vi "Get Game Time.vi"(5 "update ui":bool, 7 "Time":refnum<vi>, 8 "error in (no error)":errorcluster, 9 "Pause/Resume":bool, 11 "Application in":refnum<class "Application.lvclass">) -> (0 "error out":errorcluster, 1 "Elapsed":u32, 3 "Stringed Timer Out":string)   [LabVIEW 2021, in "Application.lvclass"]
uses:
  Application.lvclass
  Application.lvclass/Application.ctl
  <userlib>/_OpenG.lib/boolean/boolean.llb/openg_boolean__ogtk.lvlib
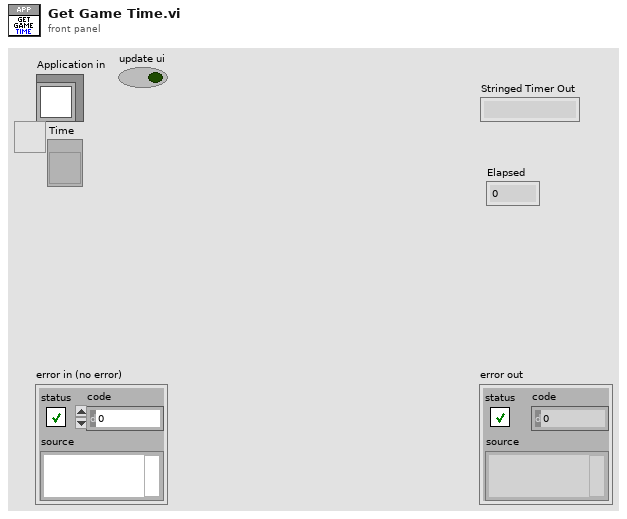
[diagram p1: front panel]
types:
  T1 = cluster{"millisecond timer value":u32, "Elapsed":u32}
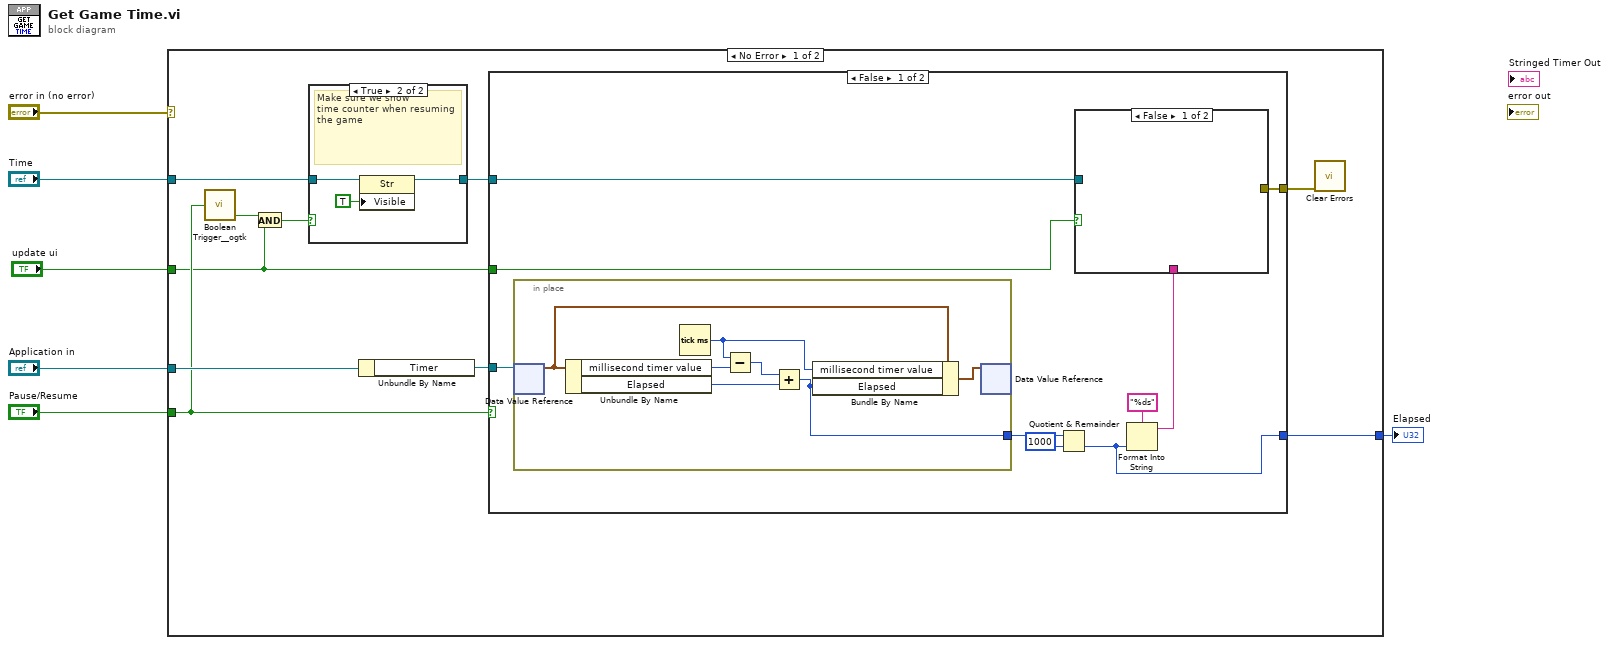
[diagram p0: block diagram]
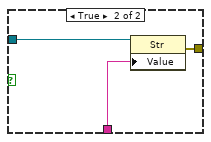
[diagram p3: hidden frame]
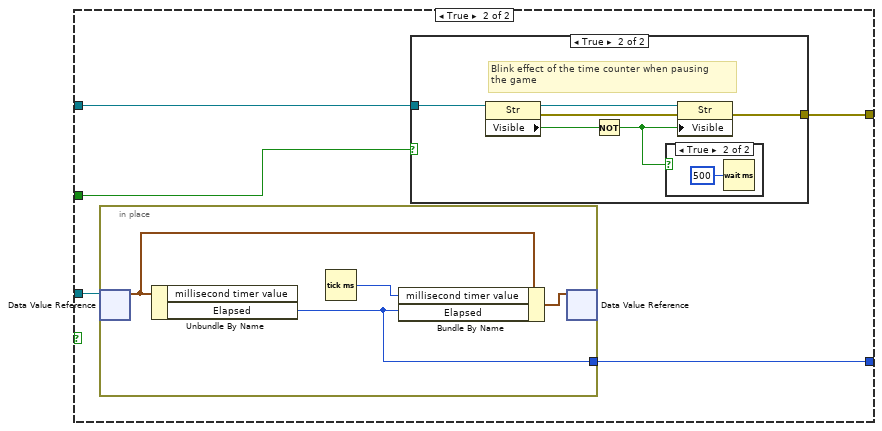
[diagram p4: hidden frame]
diagram:
  n1 = case shown="No Error" "error in (no error)" {
    tunnel: "Application in" -> [w16 _]
    tunnel: "Pause/Resume" -> [w10 _]
    tunnel: "Time" -> [w12 _]
    tunnel: [w14 _] -> w2
    tunnel: "update ui" -> [w7 _]
    frame No Error {
      n2 = call <userlib>:"Boolean Trigger__ogtk.vi"("Boolean Input"=w10) -> ("Falling Edge"=w9:bool)  [unwired: 1 in, 1 out]
      n3 = And(x=w9, y=w7) -> (x .and. y?=w8:bool)
      n4 = case shown="True" w8 {
        tunnel: w12 -> [w17 w20]
        tunnel: [w17 w19] -> w11
        frame False {
        }
        frame True {
          # "Make sure we show \ntime counter when resuming\nthe game"
          n5 = property class="Str"(reference=w20, "Visible"=TRUE) -> (reference out=w19:refnum<vi>)  [unwired: 1 in, 1 out]
        }
      }
      n6 = Unbundle By Name(w16) -> ("Timer"=w15:refnum<data-value>)
      n7 = case shown="False" w10 {
        tunnel: w15 -> [w29 w44]
        tunnel: w11 -> [w26 w43]
        tunnel: [w23 w42] -> w14
        tunnel: [w22 w41] -> w13
        tunnel: w7 -> [w21 w40]
        frame False {
          n8 = in-place {
            in-place-border: [w33] -> w25
            n9 = in-place-dvr #1(w29) -> (w36:T1)  [unwired: 1 out]
            n10 = Unbundle By Name(w36) -> ("millisecond timer value"=w39:u32, "Elapsed"=w37:u32)
            n11 = Tick Count (ms)() -> (millisecond timer value=w35:u32)
            n12 = Subtract(x=w35, y=w39) -> (x-y=w38:u32)
            n13 = Add(x=w38, y=w37) -> (x+y=w33:u32)
            n14 = Bundle By Name(cluster=w36, "millisecond timer value"=w35, "Elapsed"=w33) -> (w34:T1)
            n15 = in-place-dvr #1(w34) -> ()  [unwired: 2 out]
          }
          n16 = Quotient & Remainder(x=w25, y=u32 1000) -> (floor(x/y)=w23:u32)  [unwired: 1 out]
          n17 = Format Into String(format string="%ds", w23) -> (resulting string=w24:string)  [unwired: 2 in, 1 out]
          n18 = case shown="False" w21 {
            tunnel: w26 -> [_ w32]
            tunnel: w24 -> [_ w31]
            tunnel: [_ w30] -> w22
            frame False {
            }
            frame True {
              n19 = property class="Str"(reference=w32, "Value"=w31) -> (error out=w30:errorcluster)  [unwired: 1 in, 1 out]
            }
          }
        }
        frame True {
          n20 = in-place {
            in-place-border: [w52] -> w42
            n21 = in-place-dvr #2(w44) -> (w55:T1)  [unwired: 1 out]
            n22 = Unbundle By Name(w55) -> ("Elapsed"=w52:u32)  [unwired: 1 out]
            n23 = Tick Count (ms)() -> (millisecond timer value=w54:u32)
            n24 = Bundle By Name(cluster=w55, "millisecond timer value"=w54, "Elapsed"=w52) -> (w53:T1)
            n25 = in-place-dvr #2(w53) -> ()  [unwired: 2 out]
          }
          n26 = case shown="True" w40 {
            tunnel: w43 -> [_ w50]
            tunnel: [_ w45] -> w41
            frame False {
            }
            frame True {
              # "Blink effect of the time counter when pausing \nthe game"
              n27 = property class="Str"(reference=w50) -> (reference out=w49:refnum<vi>, error out=w46:errorcluster, "Visible"=w48:bool)  [unwired: 1 in]
              n28 = Not(x=w48) -> (.not. x?=w47:bool)
              n29 = case shown="True" w47 {
                frame False {
                }
                frame True {
                  n30 = Wait (ms)(milliseconds to wait=u32 500) -> ()  [unwired: 1 out]
                }
              }
              n31 = property class="Str"(reference=w49, error in=w46, "Visible"=w47) -> (error out=w45:errorcluster)  [unwired: 1 out]
            }
          }
        }
      }
      n32 = call <vilib>:"Clear Errors.vi"("error in (no error)"=w13) -> ()  [unwired: 5 in, 2 out]
    }
    frame Error {
    }
  }
  "Elapsed" <- w2
